vi "disdrometer.vi"(0 "Port":refnum<visa-resource-name>="Port2") -> ()   [LabVIEW 2018]
doc: "Logs and displays data in real-time from the Thies Clima Disdrometer."
uses:
  <vilib>/Platform/browser.llb/Open URL in Default Browser (path).vi
panel:
  in  "Read Period":dbl=5.0 caption="Time Target (s)"
  out "Sync Status":bool
  out "Sync String":string="Currently out of sync with Disdrometer.\nPolling at 5s delay until sync resumes."
  out "Poll Response:":string
  out "Comm String":string="\n\n\nNo response received from disdrometer.\nPlease verify connections.\n\nCommunication will be attempted again\non the rollover of the minute."
  out "Prop Logo":picture
  out "SCaN Logo":picture
  out "Observed":dbl
  in  "Debug":bool
  out "Radar Reflectivity":dbl
  out "Visibility":dbl
  in  "Filename Prefix":string="Disdrometer"
  out "Running LED":bool
  out "Uptime":string="00:00:00"
  out "Progress Bar":u32(slide) scale=0.0..60.0
  out "Date":string="2012/06/22\n12:33:20 PM"
  out "Timestamp":dbl
  out "Icon":picture
  out "Interior Temp.":dbl
  out "Observed":dbl
  out "Accumulation":dbl
  out "Rain Rate":dbl
  in  "Open Output":bool
  in  "stop":bool
  in  "Output Path":path=path "D:/Data/Disdrometer"
  out "Header":picture
  out "NASA Logo":picture
  out "Velocity":cluster{dbl[], "Diameter Distribution":dbl[]}(graph)
  out "Size":cluster{dbl[], "Diameter Distribution":dbl[]}(graph)
  out "Accumulation":cluster{"array":dbl[], "array":dbl[]}[](graph)
  out "Rain Rate":cluster{"array":dbl[], "array":dbl[]}[](graph)
  # "INPUT / OUTPUT SETTINGS"
  # "seconds"
  # "CONDITIONS"
  # "(last 1 minute)"
  # "mm / hr"
  # "mm"
  # "particles"
  # "total particles"
  # "°C"
  # "m"
  # "dBz"
  # "Recording"
  # "Version 2.6\nNASA Glenn Research Center\nmichael.j.zemba@nasa.gov"
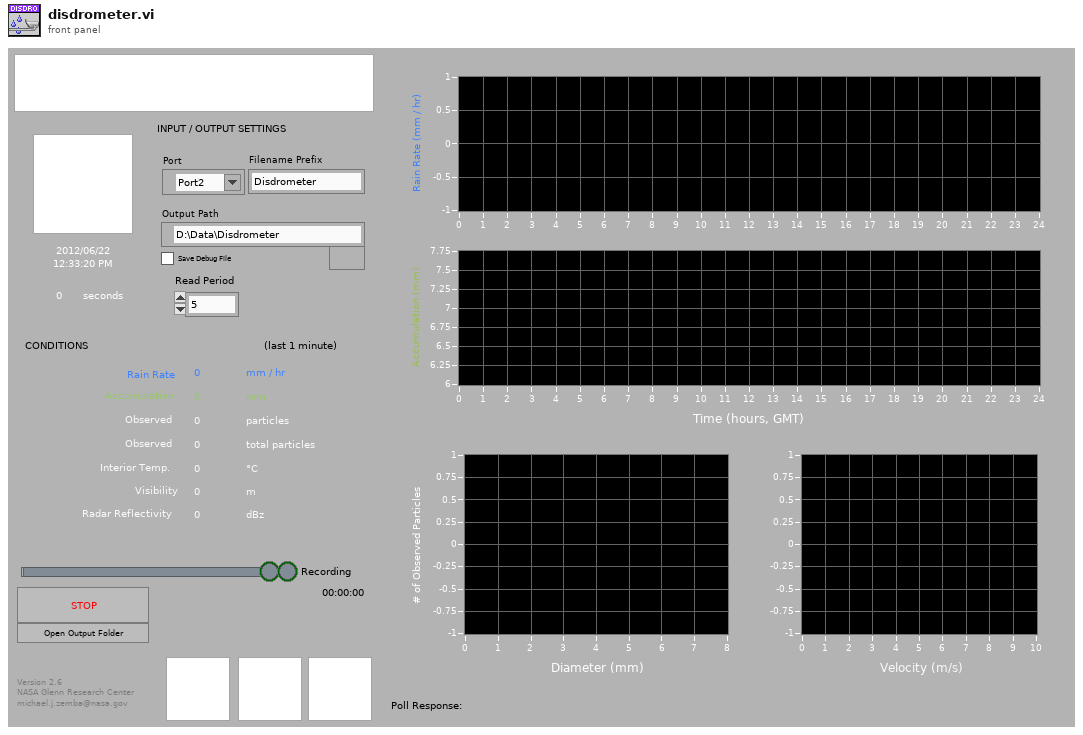
[diagram p1: front panel]
types:
  T1 = cluster{"Timestamp":dbl[], "ORG Rain Fall":dbl[]}[]
  T2 = cluster{"Timestamp":dbl[], "WXT Pressure":dbl[]}[]
  T3 = typedef "DisdromterSummaryData.ctl" = cluster{"current time":dbl, "Timestamp":dbl, "Total Rain Rate":dbl, "Liquid Rain Rate":dbl, "Solid Rain Rate":dbl, "Total Rainfall":dbl, "Visibility":dbl, "Radar Reflectivity":dbl, "Max Diameter Hail":dbl, "Measured Particles":i16, "Particle Min Speed":i16, "Particle Max Speed":i16, "Particle Min Diam":i16, "NonHydr Particles":i16, "NonHydr Volume":dbl, "Unkn Particles":i16, "Unkn Volume":dbl, "HydroType":i8}
  T4 = cluster{"[0]":dbl, "[1]":dbl, "[2]":dbl, "[3]":dbl, "[4]":dbl, "[5]":dbl}
  T5 = typedef "imagedata.ctl" = cluster{"image type":i32, "image depth":i32, "image":u8[], "mask":u8[], "colors":u32[], "Rectangle":cluster{"left":i16, "top":i16, "right":i16, "bottom":i16}}
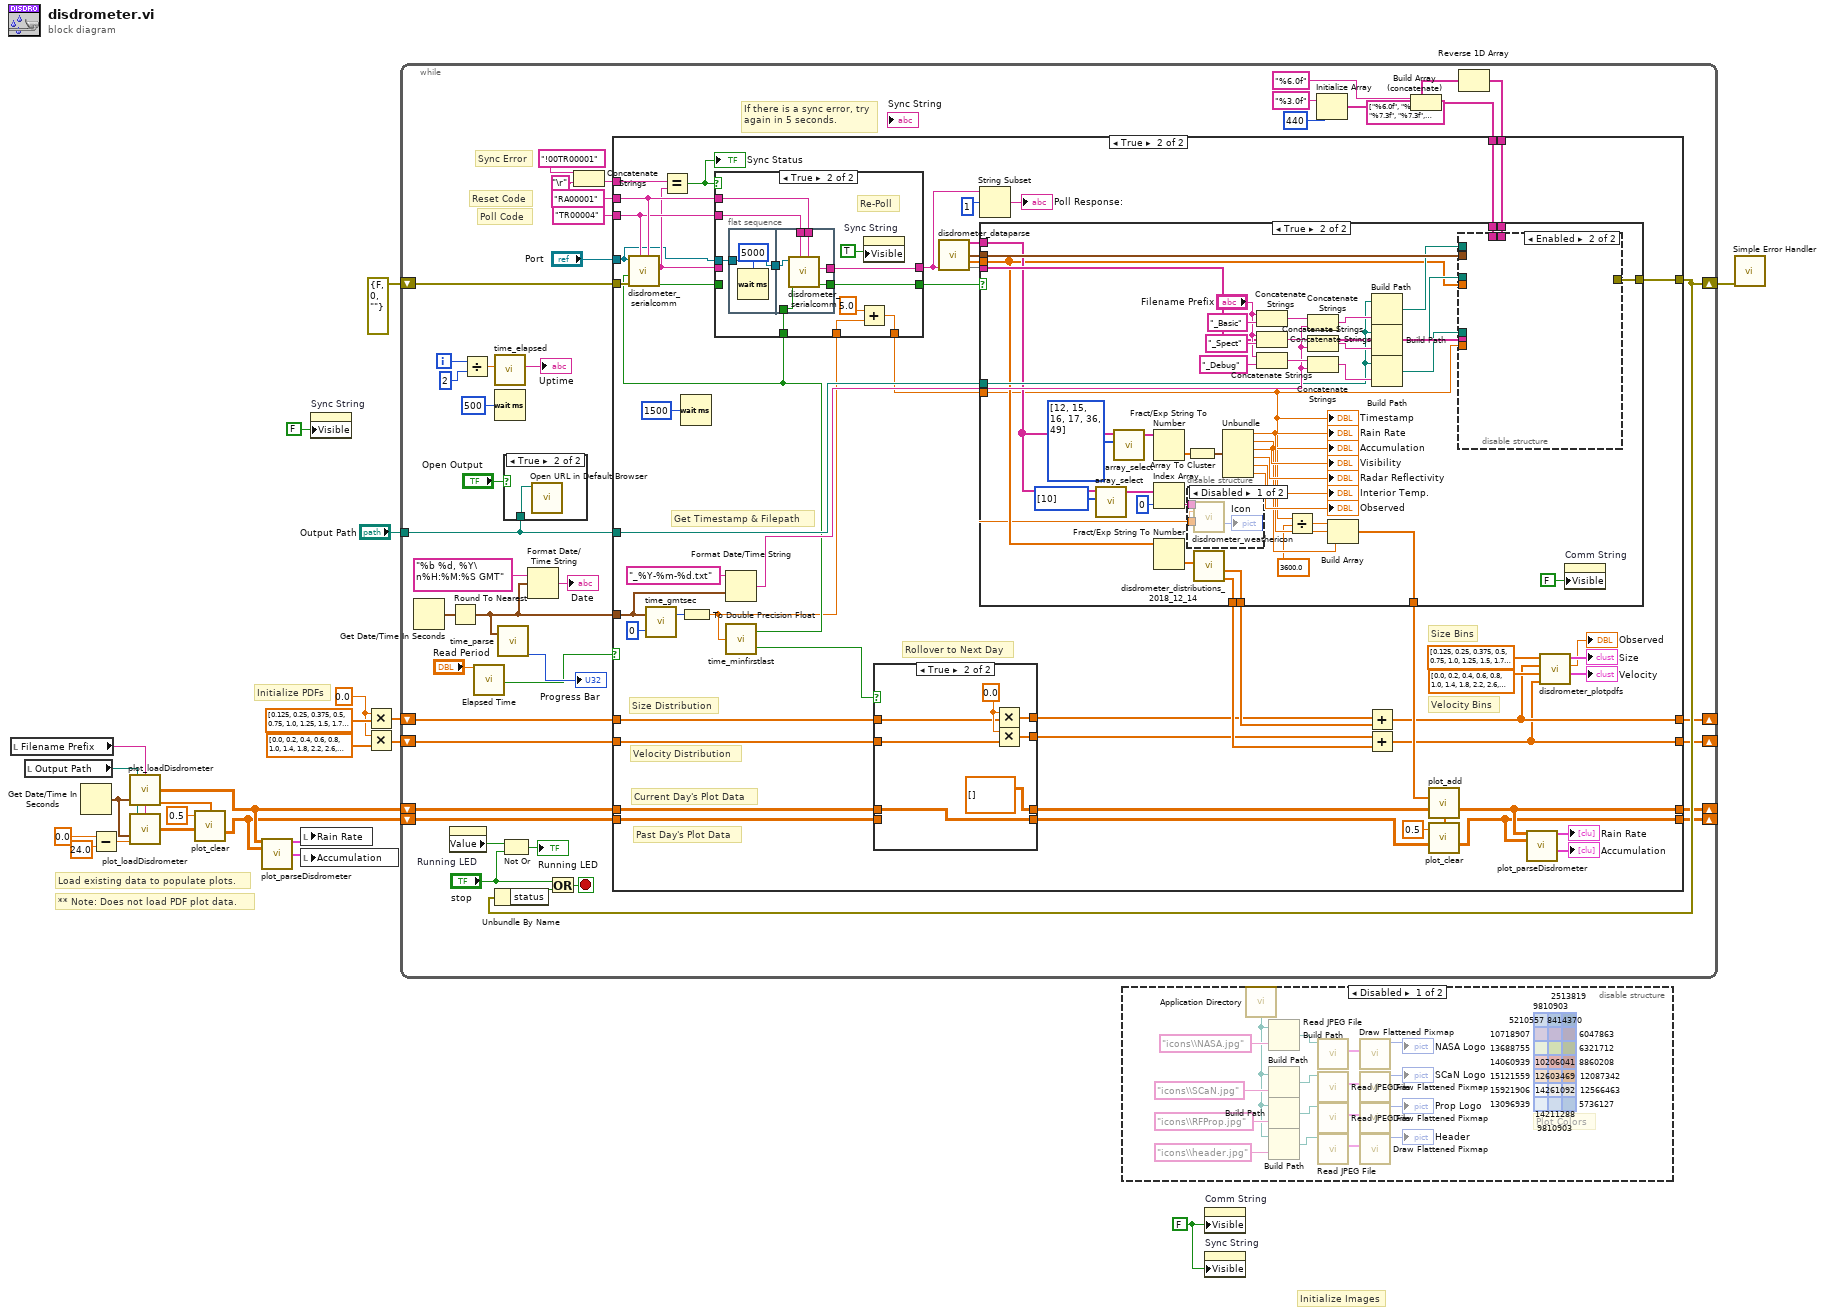
[diagram p0: block diagram]
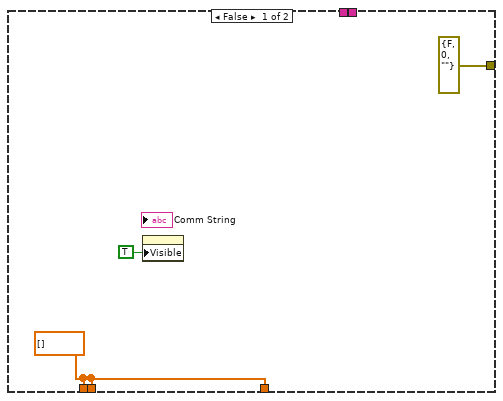
[diagram p5: hidden frame]
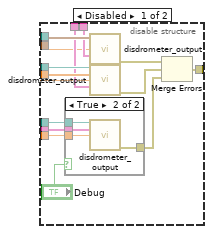
[diagram p6: hidden frame]
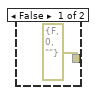
[diagram p7: hidden frame]
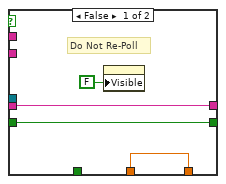
[diagram p9: hidden frame]
diagram:
  w2 = FALSE ("Visible")
  w19 = 0.0
  # "** Note: Does not load PDF plot data."
  # "Load existing data to populate plots."
  # "Initialize PDFs"
  # "Initialize Images"
  n1 = local read "Filename Prefix"() -> (w12:string)
  n2 = local read "Output Path"() -> (w11:path)
  n3 = Get Date/Time In Seconds() -> (seconds since 1Jan1904=w10:timestamp)
  n4 = Subtract(x=0.0, y=24.0) -> (x-y=w15:dbl)
  n5 = call "plot_loadDisdrometer.vi"("Output Path"=w11, "File Prefix"=w12, "Time"=w10) -> ("Loaded Data Array"=w4:dbl[][], "Timestamp"=w8:dbl[])  [unwired: 11 in]
  n6 = call "plot_loadDisdrometer.vi"("Output Path"=w11, "File Prefix"=w12, "Time"=w10, "Offset (hrs)"=w15) -> ("Loaded Data Array"=w9:dbl[][])  [unwired: 10 in, 1 out]
  n7 = call "plot_clear.vi"("Clearing Array"=w8, "Buffer Size"=0.5, "Input Arrays"=w9) -> ("Output Arrays"=w3:dbl[][])  [unwired: 12 in]
  n8 = call "plot_parseDisdrometer.vi"("Current Data"=w4, "Yesterday's Data"=w3) -> ("Plot 1"=w6:T1, "Plot 2"=w5:T2)  [unwired: 12 in]
  n9 = local write "Rain Rate"(w6) -> ()
  n10 = local write "Accumulation"(w5) -> ()
  n11 = property on="Sync String" class="Str"("Visible"=FALSE) -> ()  [unwired: 2 in, 2 out]
  n12 = Multiply(x=w19, y=dbl[] [0.125, 0.25, 0.375, 0.5, 0.75, 1.0, 1.25, 1.5, 1.75, 2.0, 2.5, 3.0, 3.5, 4.0, 4.5, 5.0, 5.5, 6.0, 6.5, 7.0, 7.5, 8.0]) -> (x*y=w17:dbl[])
  n13 = Multiply(x=w19, y=dbl[] [0.0, 0.2, 0.4, 0.6, 0.8, 1.0, 1.4, 1.8, 2.2, 2.6, 3.0, 3.4, 4.2, 5.0, 5.8, 6.6, 7.4, 8.2, 9.0, 10.0]) -> (x*y=w16:dbl[])
  n14 = while {
    tunnel: "Output Path" -> [w59]
    shift-right: [w60] -> w23
    shift-left: errorcluster {"status"=FALSE, "code"=0, "source"=""} ("error out") -> [w64]
    shift-right: [w52] -> _
    shift-left: w17 -> [w51]
    shift-right: [w50] -> _
    shift-left: w16 -> [w49]
    shift-right: [w48] -> _
    shift-left: w4 -> [w46]
    shift-right: [w47] -> _
    shift-left: w3 -> [w45]
    i -> [w41]
    stop <- w63 stop-if-true
    # "If there is a sync error, try\nagain in 5 seconds."
    # "Poll Code"
    # "Reset Code"
    # "Sync Error"
    n15 = Get Date/Time In Seconds() -> (seconds since 1Jan1904=w43:timestamp)
    n16 = Round To Nearest(number=w43) -> (nearest integer value=w42:timestamp)
    n17 = property on="Running LED" class="Bool (strict)"() -> ("Value"=w53:bool)  [unwired: 2 in, 2 out]
    n18 = Divide(x=w41, y=2) -> (x/y=w40:dbl)
    n19 = call "Elapsed Time"("Time Target (s)"="Read Period") -> ("Time has Elapsed"=w24:bool)  [unwired: 11 in, 7 out]
    n20 = call "time_elapsed.vi"("Elapsed Time (sec)"=w40) -> ("Elapsed Time (string)"=→"Uptime":string)  [unwired: 10 in]
    n21 = Wait (ms)(milliseconds to wait=u32 500) -> ()  [unwired: 1 out]
    n22 = call "time_parse.vi"("Current Time"=w42) -> ("Seconds"=→"Progress Bar":u32)  [unwired: 12 in, 6 out]
    n23 = Not Or(1:"stop", 2:w53) -> (0:→"Running LED":bool)
    n24 = case shown="True" "Open Output" {
      tunnel: w59 -> [_ w66]
      frame False {
      }
      frame True {
        n25 = call-poly <vilib>:"Open URL in Default Browser.vi"("path"=w66) -> ()  [unwired: 5 in, 2 out]
      }
    }
    n26 = Format Date/Time String(time format string (%c)="%b %d, %Y\n%H:%M:%S GMT", seconds (now)=w42) -> (date/time string=→"Date":string)  [unwired: 1 in]
    n27 = Concatenate Strings("!00TR00001" ("x"), "\r") -> (w28:string)
    n28 = Initialize Array("%3.0f", 440 ("dimension size")) -> (w36:string[])
    n29 = Build Array (concatenate)("%6.0f", w36) -> (w34:string[])
    n30 = Reverse 1D Array(array=string[] ["%6.0f", "%7.3f", "%7.3f", "%7.3f", "%7.2f", "%5.0f", "%4.1f", "%3.1f", "%5.0f", "%5.0f", "%5.0f", "%5.0f", "%5.0f", "%9.3f", "%5.0f", "%9.3f", "%5.0f", "%9.3f", "%5.0f", "%9.3f", "%5.0f", "%9.3f", "%5.0f", "%9.3f", "%5.0f", "%9.3f", "%5.0f", "%9.3f", "%5.0f", "%9.3f", "%5.0f", "%9.3f", "%5.0f", "%9.3f"] ("Format String")) -> (reversed array=w32:string[])
    n31 = case shown="True" w24 {
      tunnel: w59 -> [_ w120]
      tunnel: [w71 w119] -> w60
      tunnel: w42 -> [_ w124]
      tunnel: w64 -> [w71 w123]
      tunnel: [w70 w90] -> w52
      tunnel: w51 -> [w70 w114]
      tunnel: [w69 w89] -> w50
      tunnel: w49 -> [w69 w113]
      tunnel: [w68 w99] -> w48
      tunnel: [w67 w98] -> w47
      tunnel: w46 -> [w68 w103]
      tunnel: w45 -> [w67 w101]
      tunnel: w32 -> [_ w87]
      tunnel: w34 -> [_ w86]
      tunnel: "RA00001" ("Reset Code") -> [_ w82]
      tunnel: "TR00004" ("Poll Code") -> [_ w81]
      tunnel: "Port" -> [_ w72]
      tunnel: w28 -> [_ w75]
      frame False {
      }
      frame True {
        # "Past Day's Plot Data"
        # "Current Day's Plot Data"
        # "Velocity Bins"
        # "Size Bins"
        # "Velocity Distribution"
        # "Size Distribution"
        # "Rollover to Next Day"
        # "Get Timestamp & Filepath"
        n32 = call "time_gmtsec.vi"("Timezone Offset (Hrs)"=0, "Timestamp"=w124) -> ("Sec Since 12AM GMT"=w111:u32)  [unwired: 1 out]
        n33 = Wait (ms)(milliseconds to wait=u32 1500) -> ()  [unwired: 1 out]
        n34 = To Double Precision Float(number=w111) -> (double precision float=w80:dbl)
        n35 = Format Date/Time String(time format string (%c)="_%Y-%m-%d.txt" ("string"), seconds (now)=w124) -> (date/time string=w121:string)  [unwired: 1 in]
        n36 = call "time_minfirstlast.vi"("Sec. from Midnight"=w80) -> ("First Minute of Day"=w95:bool, "Last Minute of Day"=w83:bool)  [unwired: 2 in]
        n37 = call "disdrometer_serialcomm.vi"(5:w82, 7:w81, "Error In"=w123, 9:w83, "Resource Name"=w72) -> ("Success"=w84:bool, "Poll Response"=w74:string)  [unwired: 4 in, 1 out]
        n38 = Equal?(x=w75, y=w74) -> (x = y?=w73:bool)
        "Sync Status" <- w73
        n39 = case shown="True" w73 {
          tunnel: [w198 w208] -> w77
          tunnel: w74 -> [w198 _]
          tunnel: [w197 w207] -> w85
          tunnel: w84 -> [w197 _]
          tunnel: w83 -> [_ w209]
          tunnel: w82 -> [_ w206]
          tunnel: w81 -> [_ w205]
          tunnel: w80 -> [w196 w204]
          tunnel: [w196 w203] -> w79
          tunnel: w72 -> [_ w200]
          frame False {
            # "Do Not Re-Poll"
            n40 = property on="Sync String" class="Str"("Visible"=FALSE) -> ()  [unwired: 2 in, 2 out]
          }
          frame True {
            # "Re-Poll"
            n41 = flat-sequence {
              tunnel: [w210] -> w201
              tunnel: w200 -> [w210]
              tunnel: w209 -> [w217]
              tunnel: [w216] -> w208
              tunnel: [w215] -> w207
              tunnel: w206 -> [w214]
              tunnel: w205 -> [w213]
              tunnel: w201 -> [w212]
              frame #0 {
                n42 = Wait (ms)(milliseconds to wait=u32 5000) -> ()  [unwired: 1 out]
              }
              frame #1 {
                n43 = call "disdrometer_serialcomm.vi"(5:w214, 7:w213, 9:w217, "Resource Name"=w212) -> ("Success"=w215:bool, "Poll Response"=w216:string)  [unwired: 5 in, 1 out]
              }
            }
            n44 = Add(x=5.0, y=w204) -> (x+y=w203:dbl)
            n45 = property on="Sync String" class="Str"("Visible"=TRUE) -> ()  [unwired: 2 in, 2 out]
          }
        }
        n46 = case shown="True" w95 {
          tunnel: [w221 w227] -> w107
          tunnel: w114 -> [w221 w225]
          tunnel: [w220 w226] -> w109
          tunnel: w113 -> [w220 w224]
          tunnel: [w219 dbl[][] [] ("Output Arrays")] -> w104
          tunnel: w103 -> [w219 w222]
          tunnel: [w218 w222] -> w102
          tunnel: w101 -> [w218 _]
          frame False {
          }
          frame True {
            w228 = 0.0
            n47 = Multiply(x=w228, y=w225) -> (x*y=w227:dbl[])
            n48 = Multiply(x=w228, y=w224) -> (x*y=w226:dbl[])
          }
        }
        n49 = call "disdrometer_dataparse.vi"("Poll Response"=w77) -> ("Complete Dataset"=w116:string[], "output cluster"=w118:T3, "Spectrum Data"=w115:dbl[], 15:w117)  [unwired: 11 in]
        n50 = String Subset(string=w77, offset (0)=1) -> (substring=→"Poll Response:":string)  [unwired: 1 in]
        n51 = case shown="True" w85 {
          tunnel: w121 -> [_ w162]
          tunnel: w120 -> [_ w161]
          tunnel: [errorcluster {"status"=FALSE, "code"=0, "source"=""} ("error IO") w160] -> w119
          tunnel: w118 -> [_ w159]
          tunnel: w117 -> [_ w158]
          tunnel: w116 -> [_ w146]
          tunnel: w115 -> [_ w141]
          tunnel: [w128 w139] -> w110
          tunnel: [w128 w138] -> w108
          tunnel: [w128 w135] -> w106
          tunnel: w79 -> [_ w129]
          tunnel: w87 -> [_ w131]
          tunnel: w86 -> [_ w130]
          frame False {
            w128 = dbl[] [] ("Diameter Distribution")
            n52 = property on="Comm String" class="Str"("Visible"=TRUE) -> ()  [unwired: 2 in, 2 out]
          }
          frame True {
            n53 = call "array_select.vi"("Selection"=i32[] [10], "Array In"=w146) -> ("Array Out"=w144:string[])  [unwired: 9 in]
            n54 = call "array_select.vi"("Selection"=i32[] [12, 15, 16, 17, 36, 49], "Array In"=w146) -> ("Array Out"=w154:string[])  [unwired: 9 in]
            n55 = Fract/Exp String To Number(string=w154) -> (number=w153:dbl[])  [unwired: 3 in, 1 out]
            n56 = Index Array(array=w144, index=0) -> (element=w142:string)
            n57 = Fract/Exp String To Number(string=w141) -> (number=w140:dbl[])  [unwired: 3 in, 1 out]
            n58 = Array To Cluster(array=w153) -> (cluster=w152:T4)
            n59 = disable-structure shown="Disabled" {
              disable-tunnel: w142 -> [w193 _]
              disable-tunnel: w129 -> [w192 _]
              frame Disabled {
                n60 = call "disdrometer_weathericon.vi"("Weather Status"=w193, "Time (seconds, GMT)"=w192) -> ("Icon"=→"Icon":picture)  [unwired: 12 in, 1 out]
              }
              frame Enabled {
              }
            }
            n61 = call "disdrometer_distributions_2018_12_14.vi"("Spectrum Vector"=w140) -> ("Velocity Distribution"=w139:dbl[], "Diameter Distribution"=w138:dbl[])  [unwired: 8 in, 1 out]
            n62 = Unbundle(w152) -> ("[0]"=w137:dbl, "[1]"=w136:dbl, "[2]"=→"Visibility":dbl, "[3]"=→"Radar Reflectivity":dbl, "[4]"=→"Interior Temp.":dbl, "[5]"=→"Observed":dbl)
            "Rain Rate" <- w137
            "Accumulation" <- w136
            n63 = Concatenate Strings("Filename Prefix", "_Basic" ("string")) -> (w168:string)
            n64 = Concatenate Strings("Filename Prefix", "_Spect" ("string")) -> (w167:string)
            n65 = Concatenate Strings("Filename Prefix", "_Debug" ("string")) -> (w166:string)
            n66 = Divide(x=w129, y=3600.0) -> (x/y=w134:dbl)
            n67 = Concatenate Strings(w168, w162) -> (w165:string)
            n68 = Concatenate Strings(w167, w162) -> (w164:string)
            n69 = Concatenate Strings(w166, w162) -> (w163:string)
            n70 = Build Array(w134, w137, w136) -> (w135:dbl[])
            n71 = Build Path(base path=w161, name or relative path=w165) -> (appended path=w157:path)
            n72 = Build Path(base path=w161, name or relative path=w164) -> (appended path=w156:path)
            n73 = Build Path(base path=w161, name or relative path=w163) -> (appended path=w155:path)
            n74 = disable-structure shown="Enabled" {
              disable-tunnel: [w186 _] -> w160
              disable-tunnel: w159 -> [w185 _]
              disable-tunnel: w158 -> [w184 _]
              disable-tunnel: w157 -> [w183 _]
              disable-tunnel: w156 -> [w182 _]
              disable-tunnel: w155 -> [w181 _]
              disable-tunnel: w141 -> [w180 _]
              disable-tunnel: w131 -> [w175 _]
              disable-tunnel: w130 -> [w174 _]
              disable-tunnel: w129 -> [w173 _]
              frame Disabled {
                n75 = case shown="True" "Debug" {
                  tunnel: [errorcluster {"status"=FALSE, "code"=0, "source"=""} ("Error Out") w188] -> w178
                  tunnel: w184 -> [_ w191]
                  tunnel: w181 -> [_ w190]
                  tunnel: w173 -> [_ w189]
                  frame False {
                  }
                  frame True {
                    n76 = call "disdrometer_output.vi"("Filepath"=w190, "Data Array"=w191, "Timestamp"=w189) -> ("Error Out"=w188:errorcluster)  [unwired: 12 in]
                  }
                }
                n77 = call "disdrometer_output.vi"("Filepath"=w183, "Data Array"=w185, "Timestamp"=w173, "Format String"=w175) -> ("Error Out"=w177:errorcluster)  [unwired: 11 in]
                n78 = call "disdrometer_output.vi"("Filepath"=w182, "Data Array"=w180, "Timestamp"=w173, "Format String"=w174) -> ("Error Out"=w176:errorcluster)  [unwired: 11 in]
                n79 = Merge Errors(w177, w176, w178) -> (w186:errorcluster)
              }
              frame Enabled {
              }
            }
            n80 = property on="Comm String" class="Str"("Visible"=FALSE) -> ()  [unwired: 2 in, 2 out]
            "Timestamp" <- w129
          }
        }
        n81 = Add(x=w107, y=w108) -> (x+y=w90:dbl[])
        n82 = Add(x=w109, y=w110) -> (x+y=w89:dbl[])
        n83 = call "plot_add.vi"("Input Points"=w106, "Input Arrays"=w104) -> ("Output Arrays"=w99:dbl[][], "Timestamps"=w105:dbl[])  [unwired: 12 in]
        n84 = call "plot_clear.vi"("Clearing Array"=w105, "Buffer Size"=0.5, "Input Arrays"=w102) -> ("Output Arrays"=w98:dbl[][])  [unwired: 12 in]
        n85 = call "plot_parseDisdrometer.vi"("Current Data"=w99, "Yesterday's Data"=w98) -> ("Plot 1"=→"Rain Rate":T1, "Plot 2"=→"Accumulation":T2)  [unwired: 12 in]
        n86 = call "disdrometer_plotpdfs.vi"("Data B"=w89, "Bins B"=dbl[] [0.0, 0.2, 0.4, 0.6, 0.8, 1.0, 1.4, 1.8, 2.2, 2.6, 3.0, 3.4, 4.2, 5.0, 5.8, 6.6, 7.4, 8.2, 9.0, 10.0], "Data A"=w90, "Bins A"=dbl[] [0.125, 0.25, 0.375, 0.5, 0.75, 1.0, 1.25, 1.5, 1.75, 2.0, 2.5, 3.0, 3.5, 4.0, 4.5, 5.0, 5.5, 6.0, 6.5, 7.0, 7.5, 8.0]) -> ("PDF B"=→"Velocity":cluster{dbl[], dbl[]}, "Na"=→"Observed":dbl, "PDF A"=→"Size":cluster{dbl[], dbl[]})  [unwired: 4 in, 1 out]
      }
    }
    n87 = Unbundle By Name(w60) -> ("status"=w62:bool)
    n88 = Or(x="stop", y=w62) -> (x .or. y?=w63:bool)
  }
  n89 = disable-structure shown="Disabled" {
    frame Disabled {
      (unwired) u32 6321712
      (unwired) u32 8860208
      (unwired) u32 12087342
      (unwired) u32 12566463
      (unwired) u32 5736127
      (unwired) u32 14060939
      (unwired) u32 15121559
      (unwired) u32 15921906
      (unwired) u32 13096939
      (unwired) u32 13688755
      (unwired) u32 6047863
      (unwired) u32 10718907
      (unwired) u32 9810903
      (unwired) u32 10206041
      (unwired) u32 8414370
      (unwired) u32 12603469
      (unwired) u32 14261092
      (unwired) u32 14211288
      (unwired) u32 9810903
      (unwired) u32 2513819
      (unwired) u32 5210557
      # "Plot Colors"
      n90 = call <vilib>:"Application Directory.vi"() -> ("Application Directory"=w229:path)
      n91 = Build Path(base path=w229, name or relative path="icons\\NASA.jpg") -> (appended path=w240:path)
      n92 = Build Path(base path=w229, name or relative path="icons\\SCaN.jpg") -> (appended path=w239:path)
      n93 = Build Path(base path=w229, name or relative path="icons\\RFProp.jpg") -> (appended path=w236:path)
      n94 = Build Path(base path=w229, name or relative path="icons\\header.jpg") -> (appended path=w230:path)
      n95 = call <vilib>:"Read JPEG File.vi"("path to JPEG file"=w240) -> ("image data"=w244:T5)  [unwired: 8 in, 2 out]
      n96 = call <vilib>:"Read JPEG File.vi"("path to JPEG file"=w239) -> ("image data"=w243:T5)  [unwired: 8 in, 2 out]
      n97 = call <vilib>:"Read JPEG File.vi"("path to JPEG file"=w236) -> ("image data"=w238:T5)  [unwired: 8 in, 2 out]
      n98 = call <vilib>:"Read JPEG File.vi"("path to JPEG file"=w230) -> ("image data"=w235:T5)  [unwired: 8 in, 2 out]
      n99 = call <vilib>:"Draw Flattened Pixmap.vi"("image data"=w244) -> ("new picture"=→"NASA Logo":picture)  [unwired: 8 in]
      n100 = call <vilib>:"Draw Flattened Pixmap.vi"("image data"=w243) -> ("new picture"=→"SCaN Logo":picture)  [unwired: 8 in]
      n101 = call <vilib>:"Draw Flattened Pixmap.vi"("image data"=w238) -> ("new picture"=→"Prop Logo":picture)  [unwired: 8 in]
      n102 = call <vilib>:"Draw Flattened Pixmap.vi"("image data"=w235) -> ("new picture"=→"Header":picture)  [unwired: 8 in]
    }
    frame Enabled {
    }
  }
  n103 = property on="Comm String" class="Str"("Visible"=w2) -> ()  [unwired: 2 in, 2 out]
  n104 = property on="Sync String" class="Str"("Visible"=w2) -> ()  [unwired: 2 in, 2 out]
  n105 = call <vilib>:"Simple Error Handler.vi"("error in (no error)"=w23) -> ()  [unwired: 1 in, 8 out]
